vi "Joystick with Image Update.vi"(8 "error in (no error)":errorcluster, 9 "Camera Name":string, 10 "Image In":T1, 11 "Gantry Class in":refnum<class "Gantry.lvclass">) -> (0 "error out":errorcluster, 2 "Image Out":T1, 3 "Gantry Class out":refnum<class "Gantry.lvclass">)   [LabVIEW 2026, in "Gantry.lvclass"]
uses:
  Gantry.lvclass
  <vilib>/vision/Image Controls.llb/IMAQ Image.ctl
  <instrlib>/Aerotech Automation1/Aerotech Automation1.lvlib
panel:
  in  "stop":bool
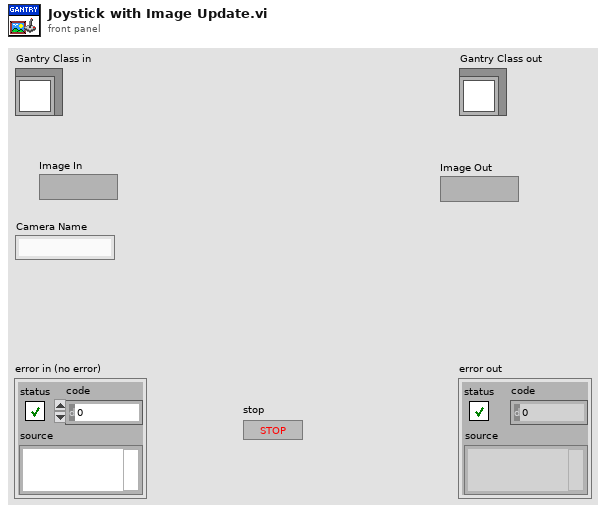
[diagram p1: front panel]
types:
  T1 = typedef "IMAQ Image.ctl" = refnum<image>
  T2 = typedef "Virtual Modes.ctl" = enum16{"Nonvirtual", "Virtual"}
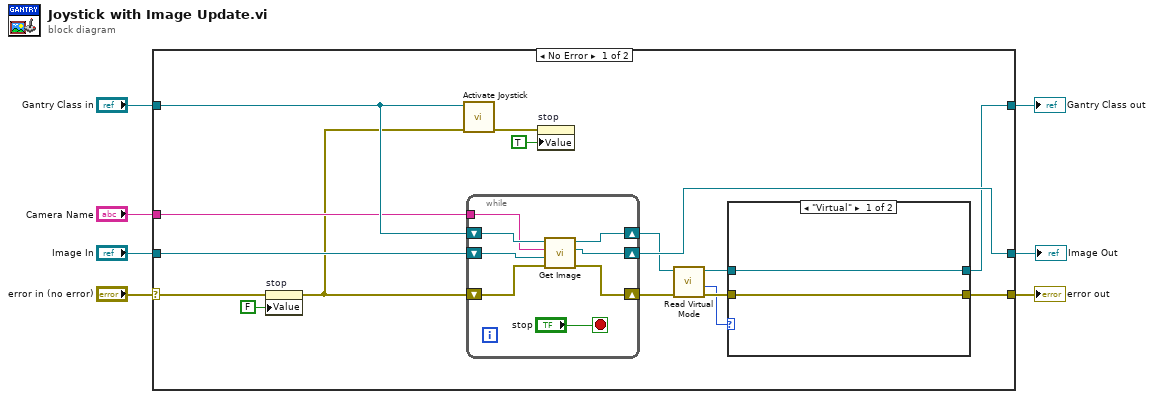
[diagram p0: block diagram]
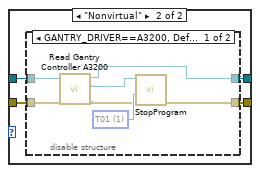
[diagram p2: hidden frame]
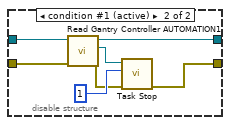
[diagram p3: hidden frame]
diagram:
  n1 = case shown="No Error" "error in (no error)" {
    selector: "error in (no error)" -> [w18 w54]
    tunnel: [w19 w54] -> w6
    tunnel: [w8 w53] -> w4
    tunnel: "Gantry Class in" -> [w21 w53]
    tunnel: "Image In" -> [w20 w52]
    tunnel: [w16 w52] -> w2
    tunnel: "Camera Name" -> [w15 _]
    frame No Error {
      n2 = property on="stop" class="Bool (strict)"(error in=w18, "Value"=FALSE) -> (error out=w14:errorcluster)  [unwired: 1 in, 1 out]
      n3 = call-dynamic "Activate Joystick.vi"("error in (no error)"=w14, "Gantry Class in"=w21) -> ("error out"=w22:errorcluster)  [unwired: 8 in, 1 out]
      n4 = while {
        shift-right: [w47] -> w12
        shift-left: w14 -> [w49]
        shift-right: [w46] -> w13
        shift-left: w21 -> [w50]
        shift-right: [w45] -> w16
        shift-left: w20 -> [w48]
        tunnel: w15 -> [w44]
        stop <- "stop" stop-if-true
        n5 = call-dynamic "Get Image.vi"("error in"=w49, "Image In"=w48, "Camera Name"=w44, "Gantry in"=w50) -> ("error out"=w47:errorcluster, "Image Out"=w45:T1, "Gantry out"=w46:refnum<class "Gantry.lvclass">)  [unwired: 4 in, 1 out]
      }
      n6 = property on="stop" class="Bool (strict)"(error in=w22, "Value"=TRUE ("stop")) -> ()  [unwired: 1 in, 2 out]
      n7 = call-dynamic "Read Virtual Mode.vi"("error in (no error)"=w12, "Gantry in"=w13) -> ("error out"=w11:errorcluster, "Virtual Mode"=w10:T2, "Gantry out"=w9:refnum<class "Gantry.lvclass">)  [unwired: 6 in, 1 out]
      n8 = case shown="\"Virtual\"" w10 {
        tunnel: [w25 w29] -> w19
        tunnel: w11 -> [w25 w26]
        tunnel: w9 -> [w24 w28]
        tunnel: [w24 w27] -> w8
        frame "Virtual" {
        }
        frame "Nonvirtual" {
          n9 = disable-structure shown="GANTRY_DRIVER==A3200, Default" {
            disable-tunnel: [w35 w37] -> w29
            disable-tunnel: w28 -> [w34 w39]
            disable-tunnel: [w31 w38] -> w27
            disable-tunnel: w26 -> [w30 w40]
            frame condition #0 {
              w36 = 1 items=["TLibrary", "T01", "T02", "T03", "T04", "T05", "T06", "T07", "T08", "T09", "T10", "T11", "T12", "T13", "T14", "T15", "T16", "T17", "T18", "T19", "T20", "T21", "T22", "T23", "T24", "T25", "T26", "T27", "T28", "T29", "T30", "T31"] ("taskId")
              n10 = call "Read Gantry Controller A3200.vi"("error in (no error)"=w30, "Gantry in"=w34) -> ("error out"=w32:errorcluster, "A3200 controller out"=w33:refnum<k24>, "Gantry out"=w31:refnum<class "Gantry.lvclass">)  [unwired: 7 in]
              n11 = call "StopProgram.vi"("error in (no error)"=w32, "taskId"=w36, "controller in"=w33) -> ("error out"=w35:errorcluster)  [unwired: 7 in, 1 out]
            }
            frame condition #1 (active) {
              n12 = call "Read Gantry Controller AUTOMATION1.vi"("error in (no error)"=w40, "Gantry in"=w39) -> ("error out"=w41:errorcluster, "Controller AUTOMATION1"=w43:refnum<k24>, "Gantry out"=w38:refnum<class "Gantry.lvclass">)  [unwired: 7 in]
              n13 = call <instrlib>:"Task Stop.vi"("error in (no error)"=w41, "Task Index"=1, "Controller Refnum"=w43) -> ("error out"=w37:errorcluster)  [unwired: 7 in, 1 out]
            }
          }
        }
      }
    }
    frame Error {
    }
  }
  "error out" <- w6
  "Gantry Class out" <- w4
  "Image Out" <- w2
